vi "LightSheetController_Test.vi"() -> ()   [LabVIEW 2018]
uses:
  <vilib>/DAQmx/configure/timing.llb/DAQmx Timing (Sample Clock).vi
  <vilib>/Waveform/WDTOps.llb/WDT Append Waveforms DBL.vi
  <resource>/objmgr/daqmx.rc
  <vilib>/DAQmx/write.llb/DAQmx Write (Analog 1D Wfm NChan NSamp).vi
  <vilib>/DAQmx/write.llb/DAQmx Write (Digital 1D Wfm NChan NSamp).vi
  <vilib>/DAQmx/create/channels.llb/DAQmx Create Channel (AO-Voltage-Basic).vi
  <vilib>/Waveform/DWDTOps.llb/DWDT Append Digital Samples.vi
  <vilib>/DAQmx/create/channels.llb/DAQmx Create Channel (DO-Digital Output).vi
panel:
  out "Graph":cluster{waveform(dbl)[], digitalwaveform[]}(graph)
  out "AnaglogWaveform":waveform(dbl)[](graph)
  out "DigitalWaveform":digitalwaveform[](graph)
  in  "Enum":enum16{"A A", "A B", "B B", "B A"}(ring)=enum."A B"
  in  "STOP":bool
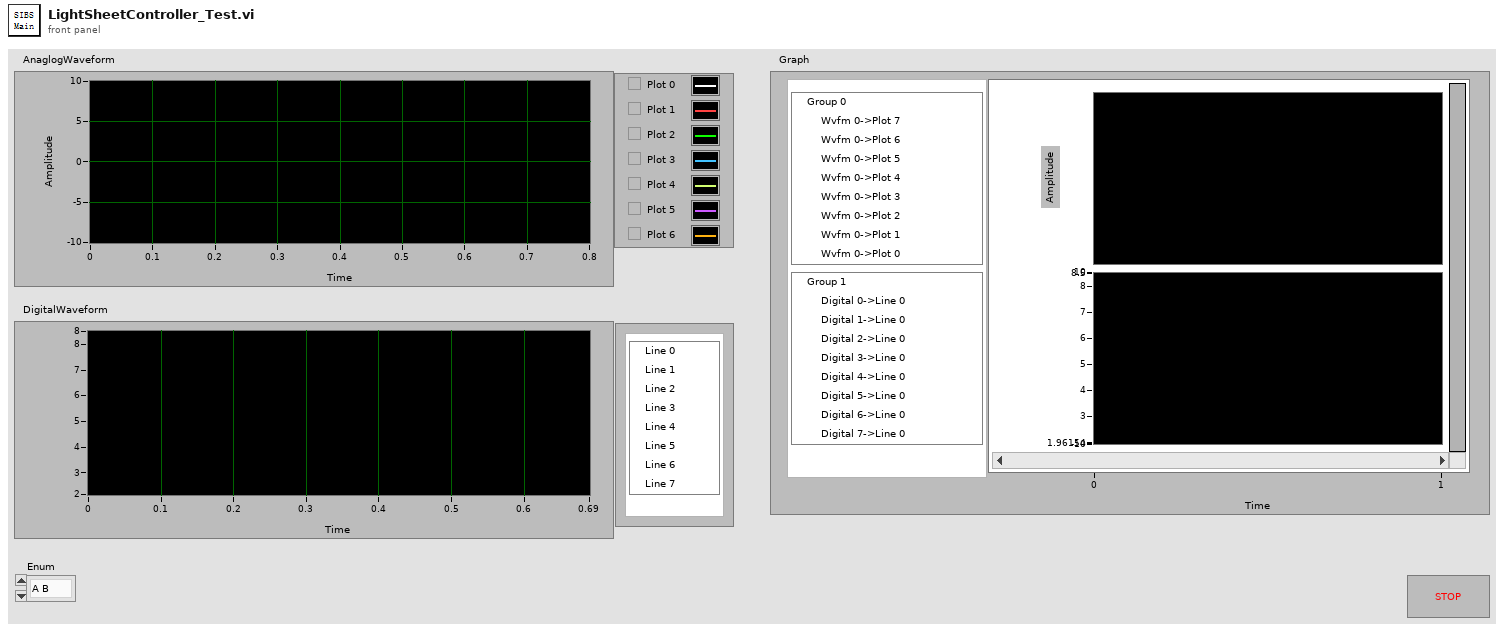
[diagram p1: front panel]
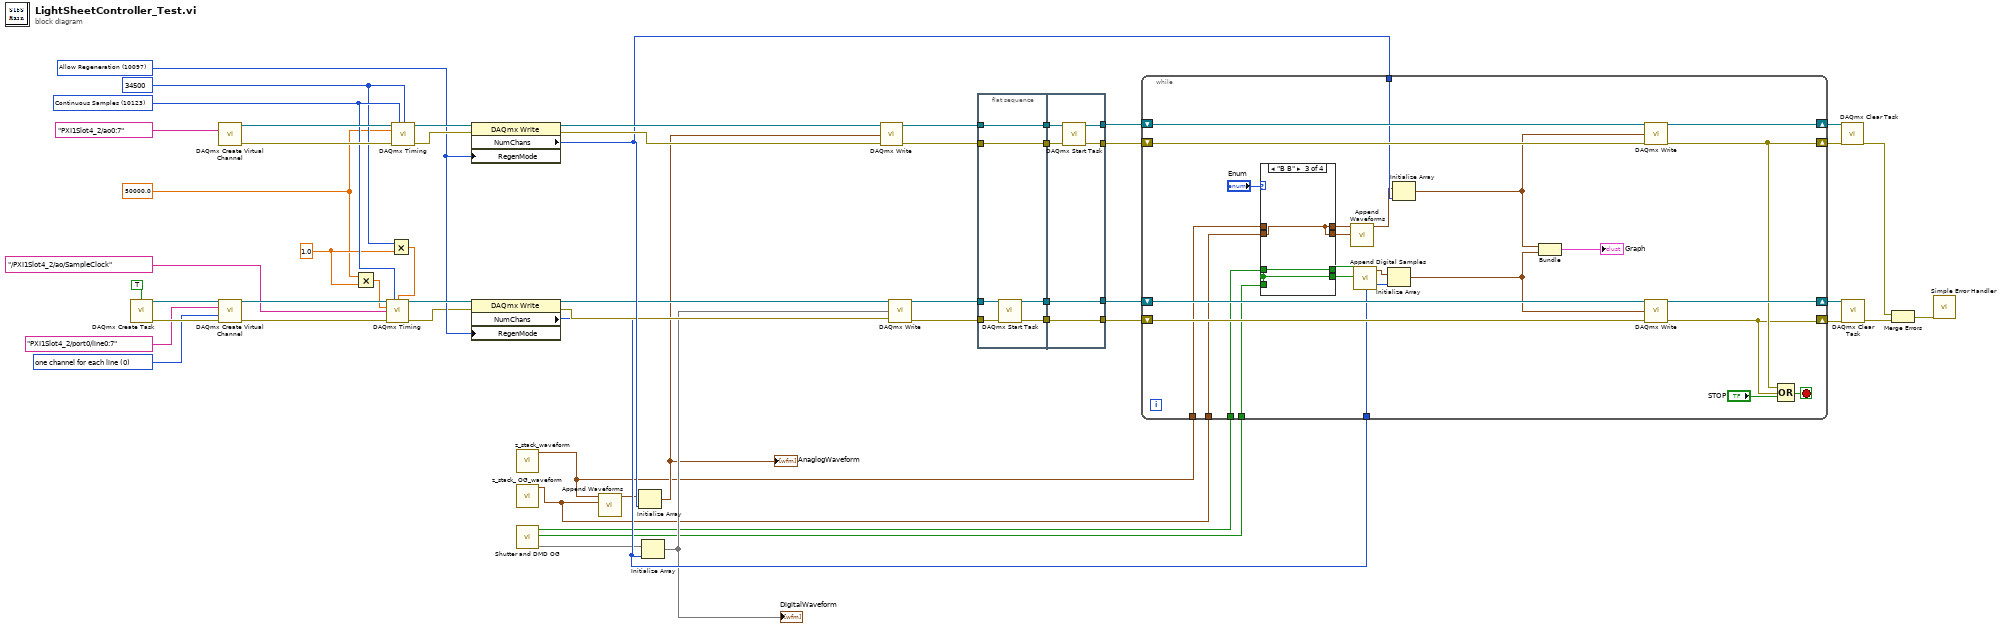
[diagram p0: block diagram]
diagram:
  w5 = 0 items=["one channel for each line", "one channel for all lines"] ("line grouping")
  w16 = 1.0 ("y")
  w19 = 10097 items=["Allow Regeneration"=10097, "Do Not Allow Regeneration"=10158] ("RegenMode")
  w18 = 34500 ("samples per channel")
  w50 = 10123 items=["Finite Samples"=10178, "Continuous Samples"=10123, "Hardware Timed Single Point"=12522] ("sample mode")
  w7 = 50000.0 ("rate")
  n1 = call <vilib>:"DAQmx Create Task.vi"("auto cleanup"=TRUE) -> ("task out"=w3:refnum<k21>, "error out"=w6:errorcluster)  [unwired: 13 in]
  n2 = call-poly <vilib>:"DAQmx Create Virtual Channel.vi"("physical channels"=tag "PXI1Slot4_2/ao0:7") -> ("task out"=w54:refnum<k21>, "error out"=w53:errorcluster)  [unwired: 13 in]
  n3 = call-poly <vilib>:"DAQmx Create Virtual Channel.vi"("task in"=w3, "lines"=tag "PXI1Slot4_2/port0/line0:7", "line grouping"=w5, "error in"=w6) -> ("task out"=w51:refnum<k21>, "error out"=w52:errorcluster)  [unwired: 10 in]
  n4 = Multiply(x=w7, y=w16) -> (x*y=w8:dbl)
  n5 = Multiply(x=w18, y=w16) -> (x*y=w17:dbl)
  n6 = call-poly <vilib>:"DAQmx Timing.vi"("task/channels in"=w51, "sample mode"=w50, "samples per channel"=w17, "rate"=w8, "source"=tag "/PXI1Slot4_2/ao/SampleClock", "error in"=w52) -> ("task out"=w24:refnum<k21>, "error out"=w1:errorcluster)  [unwired: 8 in]
  n7 = call-poly <vilib>:"DAQmx Timing.vi"("task/channels in"=w54, "sample mode"=w50, "samples per channel"=w18, "rate"=w7, "error in"=w53) -> ("task out"=w29:refnum<k21>, "error out"=w28:errorcluster)  [unwired: 9 in]
  n8 = property class="DAQmx Write"(reference=w29, error in=w28, "RegenMode"=w19) -> (reference out=w27:refnum<k21>, error out=w26:errorcluster, "NumChans"=w25:u32)
  n9 = property class="DAQmx Write"(reference=w24, error in=w1, "RegenMode"=w19) -> (reference out=w23:refnum<k21>, error out=w22:errorcluster, "NumChans"=w21:u32)
  n10 = call "z_stack_waveform.vi"() -> ("WaveformOut"=w13:waveform(dbl))  [unwired: 11 in]
  n11 = call "z_stack_ OG_waveform.vi"() -> ("waveform out"=w12:waveform(dbl))  [unwired: 15 in, 4 out]
  n12 = call "Shutter and DMD OG.vi"() -> (0:w11, "DMD OG digital output"=w9:bool[], "Shutter OG digital output"=w10:bool[])  [unwired: 8 in]
  n13 = call-poly <vilib>:"Append Waveforms.vi"("waveform B"=w12, "waveform A"=w13) -> ("waveform out"=w14:waveform(dbl))  [unwired: 8 in, 1 out]
  n14 = Initialize Array(w14, w25) -> (w15:waveform(dbl)[])
  "AnaglogWaveform" <- w15
  n15 = Initialize Array(w11, w21) -> (w20:void[])
  "DigitalWaveform" <- w20
  n16 = call-poly <vilib>:"DAQmx Write.vi"("task/channels in"=w27, "data"=w15, "error in"=w26) -> ("task out"=w48:refnum<k21>, "error out"=w44:errorcluster)  [unwired: 10 in, 1 out]
  n17 = call-poly <vilib>:"DAQmx Write.vi"("task/channels in"=w23, "data"=w20, "error in"=w22) -> ("task out"=w31:refnum<k21>, "error out"=w30:errorcluster)  [unwired: 10 in, 1 out]
  n18 = flat-sequence {
    tunnel: w48 -> [w61]
    tunnel: w31 -> [w60]
    tunnel: w30 -> [w59]
    tunnel: [w61] -> w47
    tunnel: [w58] -> w46
    tunnel: [w57] -> w45
    tunnel: w44 -> [w56]
    tunnel: [w56] -> w43
    tunnel: w47 -> [w65]
    tunnel: [w67] -> w40
    tunnel: w46 -> [w67]
    tunnel: [w66] -> w39
    tunnel: w45 -> [w66]
    tunnel: [w64] -> w42
    tunnel: w43 -> [w63]
    tunnel: [w62] -> w41
    frame #0 {
      n19 = call <vilib>:"DAQmx Start Task.vi"("task/channels in"=w60, "error in"=w59) -> ("task out"=w58:refnum<k21>, "error out"=w57:errorcluster)  [unwired: 12 in]
    }
    frame #1 {
      n20 = call <vilib>:"DAQmx Start Task.vi"("task/channels in"=w65, "error in"=w63) -> ("task out"=w64:refnum<k21>, "error out"=w62:errorcluster)  [unwired: 12 in]
    }
  }
  n21 = while {
    tunnel: w13 -> [w83]
    tunnel: w12 -> [w82]
    tunnel: w10 -> [w81]
    tunnel: w9 -> [w80]
    tunnel: w25 -> [w79]
    tunnel: w21 -> [w78]
    shift-right: [w88] -> w36
    shift-left: w40 -> [w93]
    shift-right: [w86] -> w35
    shift-left: w39 -> [w92]
    shift-right: [w87] -> w37
    shift-left: w41 -> [w90]
    shift-right: [w89] -> w38
    shift-left: w42 -> [w91]
    stop <- w85 stop-if-true
    n22 = case shown="\"B B\"" "Enum" {
      tunnel: w83 -> [w95 w99 _ w104]
      tunnel: w82 -> [_ w98 w101 w105]
      tunnel: w81 -> [w94 w97 _ w102]
      tunnel: w80 -> [_ w96 w100 w103]
      tunnel: [w95 w99 w101 w105] -> w76
      tunnel: [w95 w98 w101 w104] -> w75
      tunnel: [w94 w97 w100 w103] -> w74
      tunnel: [w94 w96 w100 w102] -> w73
      frame "A A", Default {
      }
      frame "A B" {
      }
      frame "B B" {
      }
      frame "B A" {
      }
    }
    n23 = call-poly <vilib>:"Append Waveforms.vi"("waveform B"=w75, "waveform A"=w76) -> ("waveform out"=w72:waveform(dbl))  [unwired: 8 in, 1 out]
    n24 = call-poly <vilib>:"Append Digital Samples.vi"("digital waveform B"=w73, "digital waveform A"=w74) -> ("digital waveform out"=w71:digitalwaveform)  [unwired: 8 in, 1 out]
    n25 = Initialize Array(w71, w78) -> (w69:digitalwaveform[])
    n26 = Initialize Array(w72, w79) -> (w70:waveform(dbl)[])
    n27 = Bundle(w70, w69) -> (→"Graph":cluster{waveform(dbl)[], digitalwaveform[]})  [unwired: 1 in]
    n28 = call-poly <vilib>:"DAQmx Write.vi"("task/channels in"=w91, "data"=w70, "error in"=w90) -> ("task out"=w89:refnum<k21>, "error out"=w87:errorcluster)  [unwired: 10 in, 1 out]
    n29 = call-poly <vilib>:"DAQmx Write.vi"("task/channels in"=w93, "data"=w69, "error in"=w92) -> ("task out"=w88:refnum<k21>, "error out"=w86:errorcluster)  [unwired: 10 in, 1 out]
    n30 = Compound Arithmetic op=OR(w87, w86, "STOP") -> (w85:bool)
  }
  n31 = call <vilib>:"DAQmx Clear Task.vi"("task in"=w38, "error in"=w37) -> ("error out"=w34:errorcluster)  [unwired: 13 in]
  n32 = call <vilib>:"DAQmx Clear Task.vi"("task in"=w36, "error in"=w35) -> ("error out"=w33:errorcluster)  [unwired: 13 in]
  n33 = Merge Errors(w34, w33) -> (w32:errorcluster)
  n34 = call <vilib>:"Simple Error Handler.vi"("error in (no error)"=w32) -> ()  [unwired: 4 in, 5 out]
